vi "+S2C_UTILITY_Process.vi"(8 "Error In":errorcluster) -> (0 "Error Out":errorcluster)   [LabVIEW 2015]
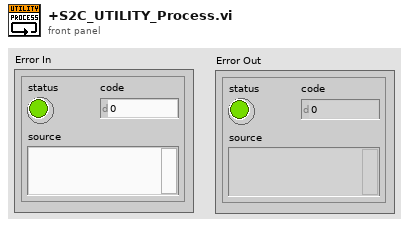
[diagram p1: front panel]
types:
  T1 = cluster{"Caller-Q":refnum<queue>, "Command":string, "Return":string, "Data":variant, "Timeout":dbl}
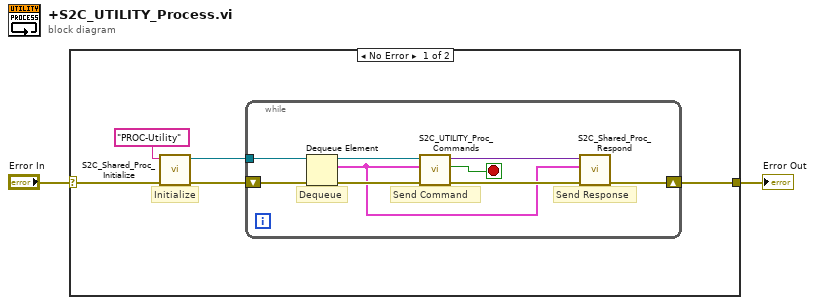
[diagram p0: block diagram]
diagram:
  n1 = case shown="No Error" "Error In" {
    selector: "Error In" -> [w6 w17]
    tunnel: [w7 w17] -> w1
    frame No Error {
      # "Initialize"
      n2 = call "S2C_Shared_Proc_Initialize.vi"("Error In"=w6, "Q-Name"="PROC-Utility" ("name (unnamed)")) -> ("Error Out"=w5:errorcluster, "Q-Ref"=w4:refnum<queue>)  [unwired: 8 in]
      n3 = while {
        shift-right: [w14] -> w7
        shift-left: w5 -> [w16]
        tunnel: w4 -> [w15]
        stop <- w10 stop-if-true
        # "Send Command"
        # "Send Response"
        # "Dequeue"
        n4 = Dequeue Element(queue=w15, error in (no error)=w16) -> (queue out=w8:refnum<queue>, element=w9:T1, error out=w13:errorcluster)  [unwired: 1 in, 1 out]
        n5 = call "S2C_UTILITY_Proc_Commands.vi"("Error In"=w13, "Settings"=w9, "Q-Ref"=w8) -> ("Error Out"=w11:errorcluster, "Stop?"=w10:bool, "Response"=w12:variant)  [unwired: 6 in]
        n6 = call "S2C_Shared_Proc_Respond.vi"("Error In"=w11, "Settings"=w9, "Response"=w12) -> ("Error Out"=w14:errorcluster)  [unwired: 8 in]
      }
    }
    frame Error {
    }
  }
  "Error Out" <- w1
